vi "Globals.vi"() -> ()   [LabVIEW 2015]
panel:
  in  "devices_amount":u8
  in  "reg_addr-CC_position":u8
  in  "cams_amount":u8
  in  "reg_addr-CH_select":u8
  in  "reg_addr-PIXEL_AMOUNT":u8
  in  "maddr of CC":u8
  in  "cam_sel":u8
  in  "nosnobchanged":bool
  in  "board_sel":u8
  in  "nob":u32
  in  "dioden 2":u16[][](array[numeric])
  in  "dioden 1":u16[][](array[numeric])
  in  "exp time":dbl
  in  "nos":u32
  in  "PIXEL":u32
  in  "boards":u32
  # "registers of CC"
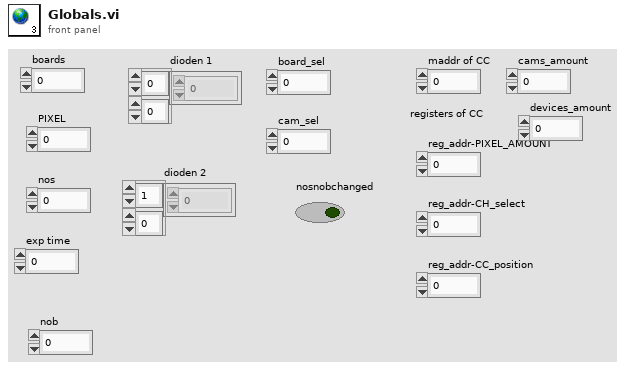
[diagram p1: front panel]
diagram:
